vi "FFT Skew Detection.vi"(8 "error in (no error)":errorcluster, 11 "Refnum In":T2) -> (0 "error out":errorcluster, 1 "Error (Degrees)":dbl format="%_6g", 2 "Error (Radians)":dbl format="%_6f", 3 "Fit Line":T2(plugin-control), 4 "Alt. Angle (Degrees)":dbl format="%_6g", 5 "Alt. Angle (Radians)":dbl format="%_6g", 6 "Angle (Degrees)":dbl format="%_6g", 7 "Angle (Radians)":dbl format="%_6g")   [LabVIEW 2016]
uses:
  <vilib>/vision/Image Controls.llb/IMAQ Image.ctl
  <vilib>/Analysis/6fits.llb/Confidence Interval (Linear).vi
  <vilib>/vision/NI_Vision_Development_Module.lvlib
  <vilib>/Analysis/6fits.llb/Curve Fitting Criteria.ctl
  <vilib>/Analysis/NI_AALPro.lvlib
panel:
  in  "Tab Control":T1(tab)
  out "Original Image":T2(plugin-control)
  in  "File Path":path=path "D:/Documents/School/Brookhaven/Images/Pixel to Micron Test/image_000_600_60_15_rotated_45_degrees.png"
  out "FFT":T2(plugin-control)
  out "Zoom":T2(plugin-control)
  in  "Image Zoom":sgl=1.0
  out "Image Center Y":u32
  out "Image Center X":u32
  out "Captured FFT Spectrum":picture
  out "Load as U8":T2(plugin-control)
  in  "Settings":T3={"Objects"=0, "Threshold"=160, "Reject Border"=TRUE, "Fill Holes"=FALSE, "Min Object Size"=FALSE, "Min Size"=2, "Max Object Size"=FALSE, "Max Size"=100, "Show Search Area"=FALSE, "Show Center"=TRUE, "Show Bounding Box"=TRUE} {"Objects" items=["Bright Objects", "Dark Objects"]; "Threshold" min=1 max=999999999 step=1; "Max Size" min=1 max=999999999 step=1; "Min Size" min=1 max=999999999 step=1}
  out "Number of Objects Found":i32
  out "Find Objects":T2(plugin-control)
  out "Image Aspect Ratio":dbl
  out "Adjusted Slope Error":dbl format="%^_4e"
  out "Adjusted Slope":dbl format="%_6g"
  out "Line Equation":cluster{"A":dbl, "B":dbl, "C":dbl} {"C" format="%_6f"; "B" format="%_6f"; "A" format="%_6f"}
  out "Valid Fit?":bool
  out "X":sgl[](array[numeric])
  out "Y":sgl[](array[numeric])
  out "IMAQ Fit Slope":dbl format="%_6g"
  out "Residual":dbl format="%.2f"
  out "IMAQ Fit Intercept":dbl
  out "IMAQ Fit Delta Slope":dbl
  out "IMAQ Fit Delta Intercept":dbl
  out "Sigma":sgl[](array[numeric])
  # "Skew Angle (0 to 180 Degrees)"
  # "Skew Angle (90 to -90 Degrees)"
  # "Error"
  # "Line Fit"
  # "Ax + By + C = 0"
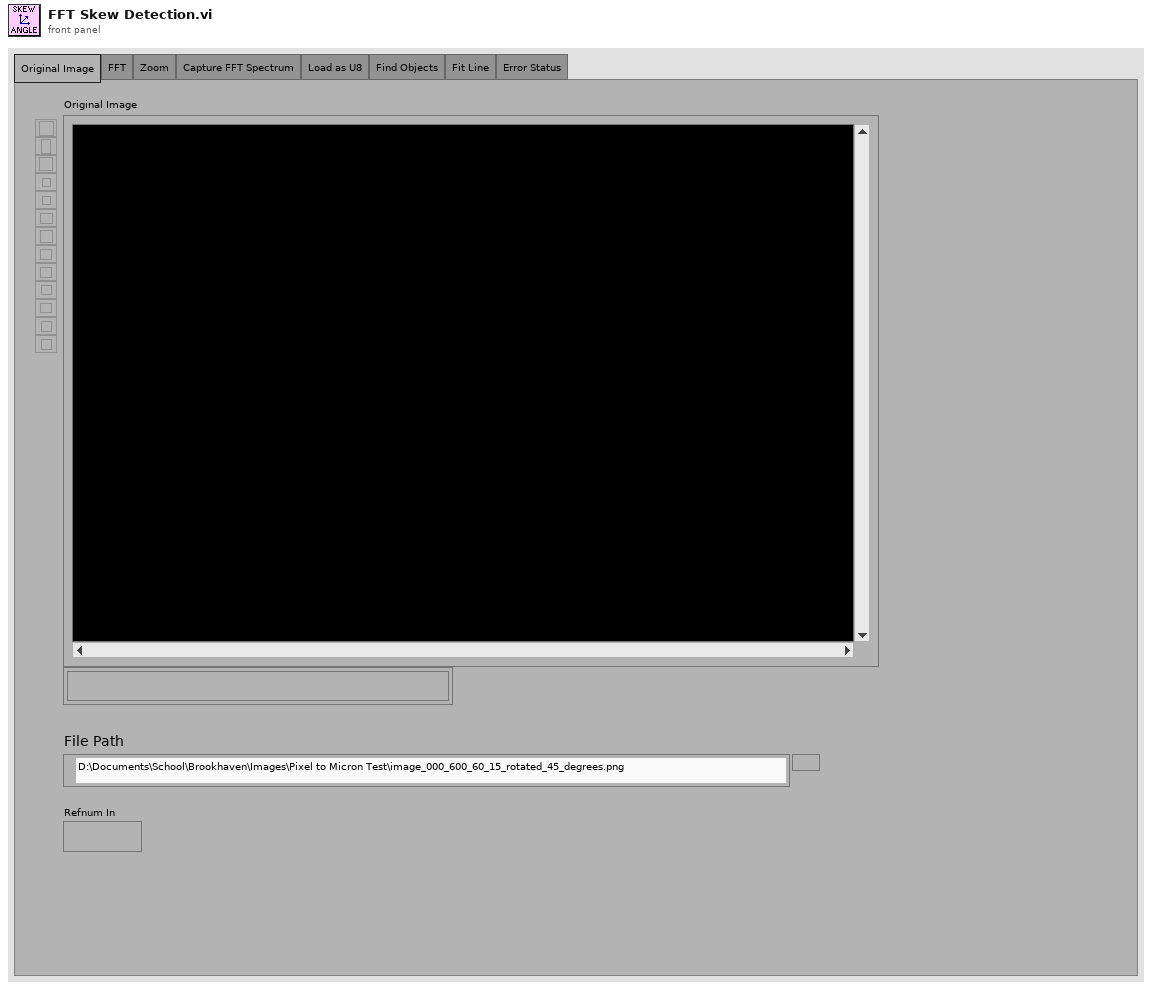
[diagram p1: front panel]
types:
  T1 = enum32{"Original Image", "FFT", "Zoom", "Capture FFT Spectrum", "Load as U8", "Find Objects", "Fit Line", "Error Status"}
  T2 = typedef "IMAQ Image.ctl" = refnum<image>
  T3 = cluster{"Objects":u16, "Threshold":i32, "Reject Border":bool, "Fill Holes":bool, "Min Object Size":bool, "Min Size":i32, "Max Object Size":bool, "Max Size":i32, "Show Search Area":bool, "Show Center":bool, "Show Bounding Box":bool}
  T4 = typedef "Image Type" = u32
  T5 = typedef "imagedata.ctl" = cluster{"image type":i32, "image depth":i32, "image":u8[], "mask":u8[], "colors":u32[], "Rectangle":cluster{"left":i16, "top":i16, "right":i16, "bottom":i16}}
  T6 = cluster{"Object Center":cluster{"X":sgl, "Y":sgl}, "Bounding Box":cluster{"X Left":i32, "Y Top":i32, "X Right":i32, "Y Bottom":i32}, "Area":sgl, "Orientation":sgl, "Aspect Ratio":sgl, "Nb Holes":i32}[]
  T7 = cluster{"Point 1":cluster{"X":sgl, "Y":sgl}, "Point 2":cluster{"X":sgl, "Y":sgl}}
  T8 = typedef "NI_AALPro.lvlib/Curve Fitting Criteria.ctl" = u16
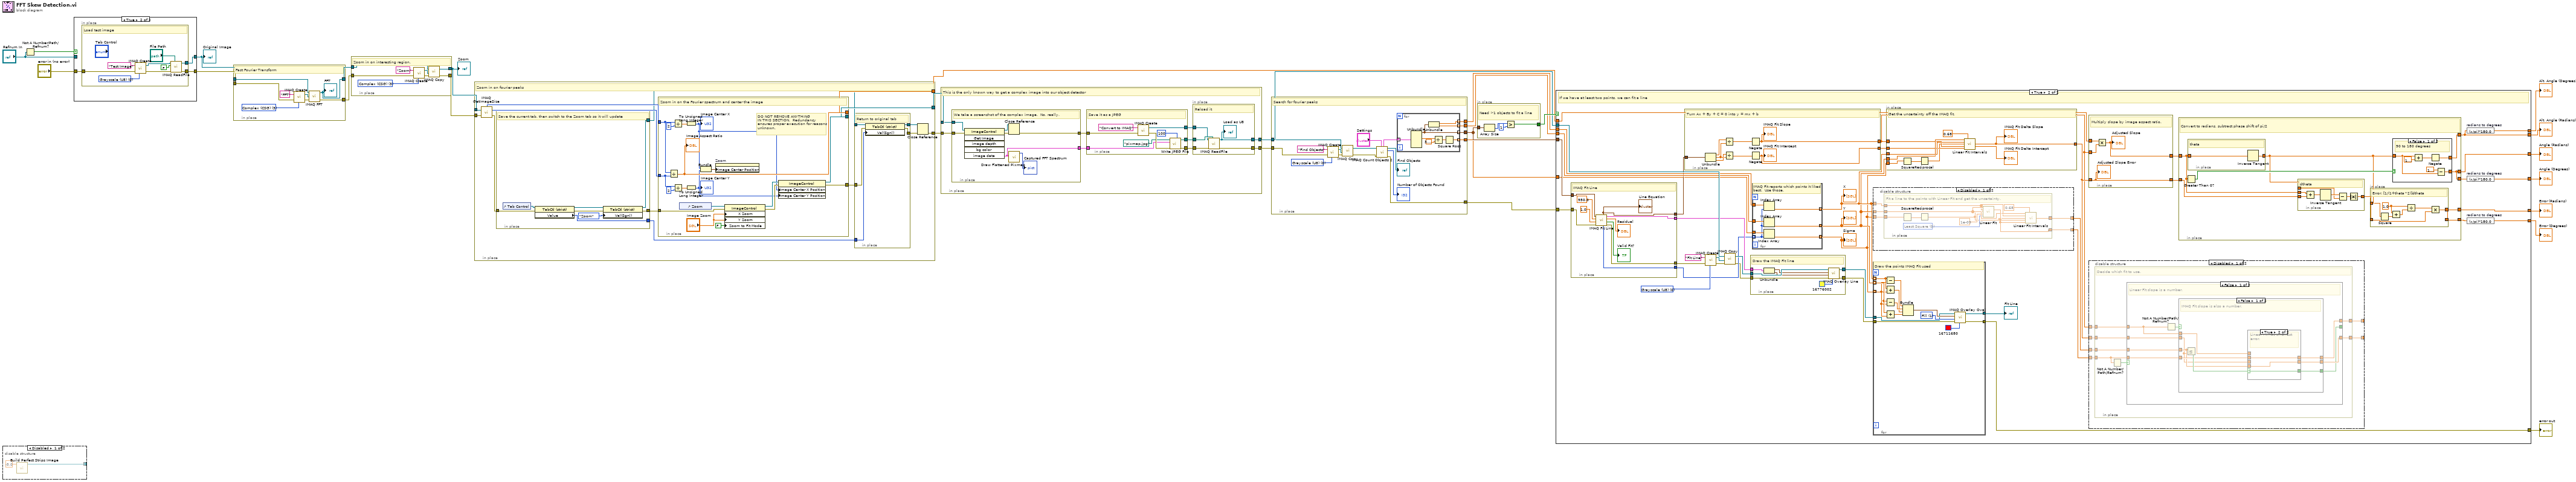
[diagram p0: block diagram]
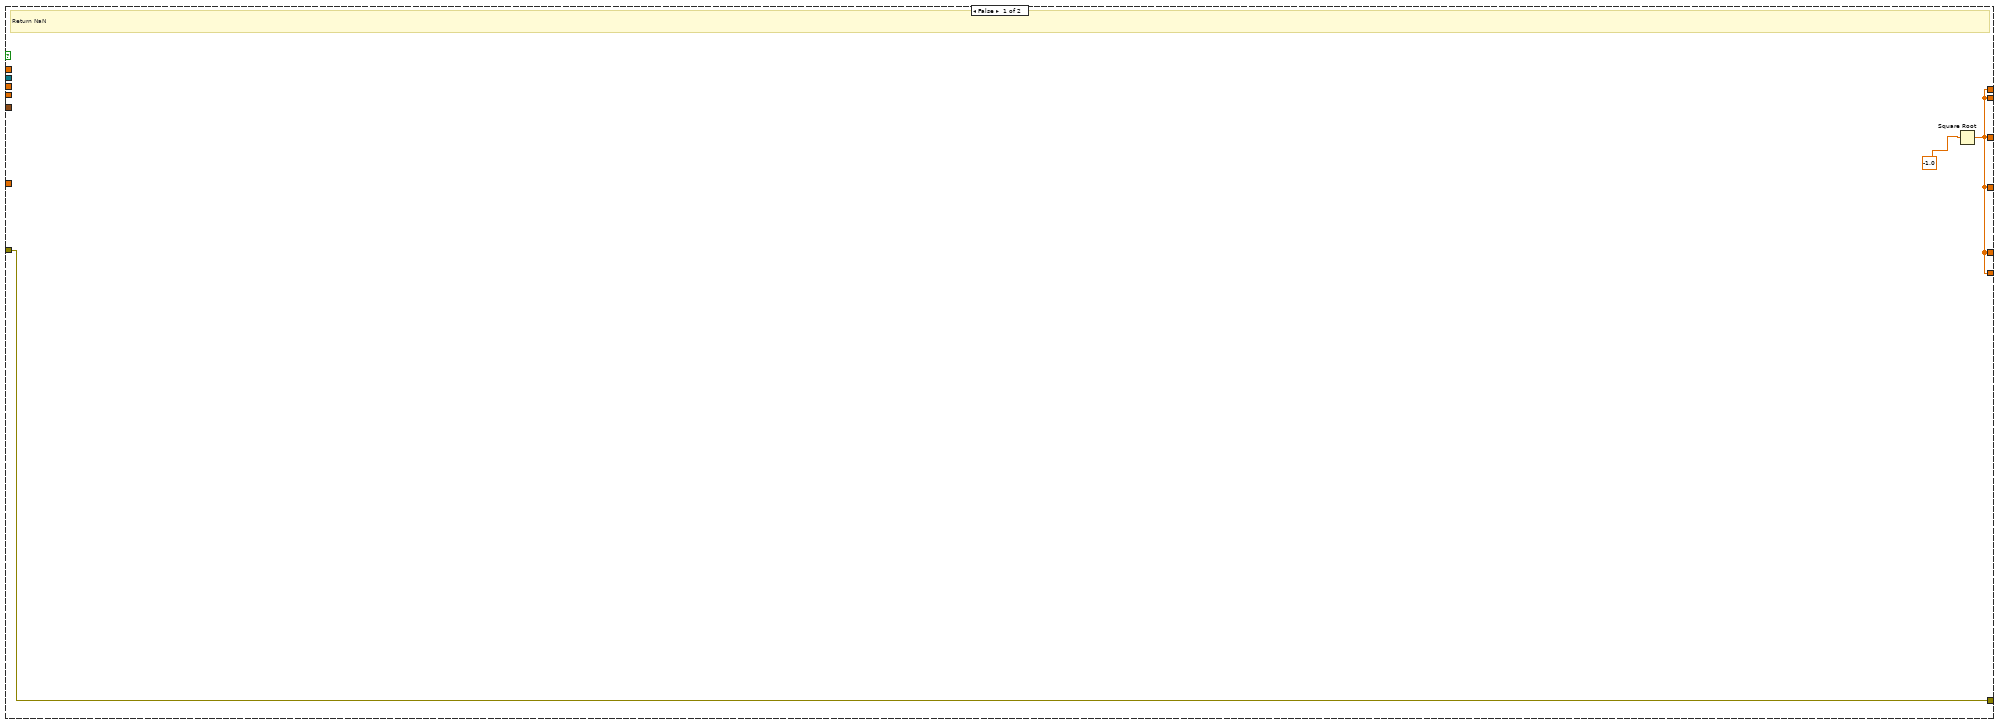
[diagram p4: hidden frame]
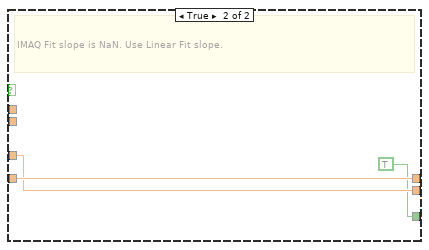
[diagram p7: hidden frame]
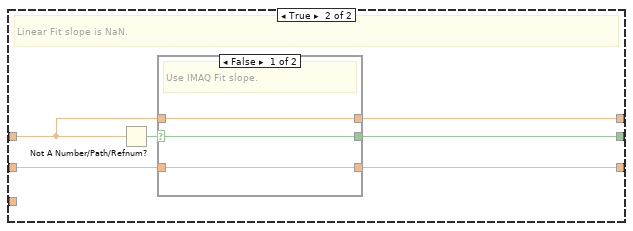
[diagram p8: hidden frame]
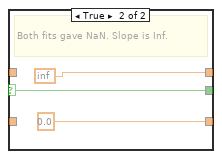
[diagram p9: hidden frame]
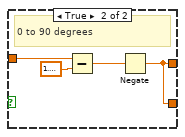
[diagram p11: hidden frame]
diagram:
  n1 = disable-structure shown="Disabled" {
    disable-tunnel: [w28 _] -> _
    frame Disabled {
      n2 = call "Build Perfect Strips Image.vi"("Angle (degrees)"=sgl -5.0) -> ("Image Out"=w28:T2)  [unwired: 9 in, 1 out]
    }
    frame Enabled {
    }
  }
  n3 = Not A Number/Path/Refnum?(number/path/refnum="Refnum In") -> (NaN/Path/Refnum?=w14:bool)
  n4 = case shown="True" w14 {
    tunnel: "error in (no error)" -> [w30 w34]
    tunnel: [w30 w33] -> w26
    tunnel: [w31 w32] -> w13
    tunnel: "Refnum In" -> [w31 _]
    frame False {
    }
    frame True {
      n5 = in-place {
        in-place-border: [w35] -> w32
        in-place-border: [w37] -> w33
        in-place-border: w34 -> [w36]
        w40 = T4 0 items=["Grayscale (U8)", "Grayscale (I16)", "Grayscale (SGL)", "Complex (CSG)", "RGB (U32)", "HSL (U32)", "RGB (U64)", "Grayscale (U16)"] ("Image Type")
        # "Load test image"
        n6 = call "IMAQ Create"("Image Name"="Test Image", "Image Type"=w40, "error in (no error)"=w36) -> ("New Image"=w41:T2, "error out"=w38:errorcluster)  [unwired: 2 in]
        n7 = call "IMAQ ReadFile"("File Path"="File Path", "error in (no error)"=w38, "Load Color Palette? (No)"=FALSE, "Image"=w41) -> ("error out"=w37:errorcluster, "Image Out"=w35:T2)  [unwired: 3 in, 3 out]
      }
    }
  }
  "Original Image" <- w13
  n8 = in-place {
    in-place-border: w26 -> [w51]
    in-place-border: w13 -> [w47]
    in-place-border: [w46] -> w22
    in-place-border: [w44] -> w8
    w49 = T4 3 items=["Grayscale (U8)", "Grayscale (I16)", "Grayscale (SGL)", "Complex (CSG)", "RGB (U32)", "HSL (U32)", "RGB (U64)", "Grayscale (U16)"] ("Image Type")
    # "Fast Fourier Transform"
    n9 = call "IMAQ Create"("Image Name"="FFT", "Image Type"=w49, "error in (no error)"=w51) -> ("New Image"=w48:T2, "error out"=w45:errorcluster)  [unwired: 2 in]
    n10 = call "IMAQ FFT"("error in (no error)"=w45, "Image Dst"=w48, "Image Src"=w47) -> ("error out"=w44:errorcluster, "Image Dst Out"=w46:T2)  [unwired: 1 in]
    "FFT" <- w46
  }
  n11 = in-place {
    in-place-border: w22 -> [w56]
    in-place-border: [w55] -> w10
    in-place-border: w8 -> [w54]
    in-place-border: [w52] -> w7
    w58 = T4 3 items=["Grayscale (U8)", "Grayscale (I16)", "Grayscale (SGL)", "Complex (CSG)", "RGB (U32)", "HSL (U32)", "RGB (U64)", "Grayscale (U16)"] ("Image Type")
    # "Zoom in on interesting region."
    n12 = call "IMAQ Create"("Image Name"="Zoom", "Image Type"=w58, "error in (no error)"=w54) -> ("New Image"=w57:T2, "error out"=w53:errorcluster)  [unwired: 2 in]
    n13 = call "IMAQ Copy"("error in (no error)"=w53, "Image Dst"=w57, "Image Src"=w56) -> ("error out"=w52:errorcluster, "Image Dst Out"=w55:T2)  [unwired: 3 in]
  }
  "Zoom" <- w10
  n14 = in-place {
    in-place-border: w10 -> [w73]
    in-place-border: [w70] -> w19
    in-place-border: [w69] -> w9
    in-place-border: w7 -> [w68]
    in-place-border: [w60] -> w6
    # "Zoom in on fourier peaks"
    n15 = call "IMAQ GetImageSize"("Image"=w73, "error in (no error)"=w68) -> ("Y Resolution"=w71:i32, "X Resolution"=w72:i32, "error out"=w66:errorcluster)  [unwired: 2 in]
    n16 = in-place {
      in-place-border: [w103] -> w67
      in-place-border: w66 -> [w101]
      in-place-border: [w98] -> w64
      in-place-border: [w97] -> w63
      # "Save the current tab, then switch to the Zoom tab so it will update"
      n17 = control-ref of="Tab Control"() -> (w102:refnum<vi>)
      n18 = property class="TabCtl (strict)"(reference=w102, error in=w101) -> (reference out=w99:refnum<vi>, error out=w100:errorcluster, "Value"=w97:T1)
      n19 = property class="TabCtl (strict)"(reference=w99, error in=w100, "Val(Sgnl)"=T1."Zoom" ("Value")) -> (reference out=w98:refnum<vi>, error out=w103:errorcluster)
    }
    n20 = in-place {
      in-place-border: w72 -> [w94]
      in-place-border: w71 -> [w93]
      in-place-border: [w92] -> w70
      in-place-border: [w87] -> w69
      in-place-border: w67 -> [w86]
      in-place-border: [w85] -> w65
      # "DO NOT REMOVE ANYTHING\nIN THIS SECTION.  Redundancy\nensures proper execution for reasons\nunknown."
      # "Zoom in on the Fourier spectrum and center the image"
      n21 = Divide(x=w94, y=w93) -> (x/y=w92:dbl)
      "Image Aspect Ratio" <- w92
      n22 = Divide(x=w94, y=2) -> (x/y=w91:dbl)
      n23 = Divide(x=w93, y=2) -> (x/y=w90:dbl)
      n24 = control-ref of="Zoom"() -> (w88:refnum<vi>)
      n25 = To Unsigned Long Integer(number=w91) -> (unsigned 32bit integer=w81:u32)
      "Image Center X" <- w81
      n26 = To Unsigned Long Integer(number=w90) -> (unsigned 32bit integer=w80:u32)
      "Image Center Y" <- w80
      n27 = Bundle(w81, w80) -> (w79:cluster{u32, u32})  [unwired: 1 in]
      n28 = property on="Zoom" class="ImageControl"("Image Center Position"=w79) -> ()  [unwired: 2 in, 2 out]
      n29 = property on="Property Node" class="ImageControl"(reference=w88, error in=w86, "X Zoom"="Image Zoom", "Y Zoom"="Image Zoom", "Zoom to Fit Mode"=FALSE) -> (reference out=w82:refnum<vi>, error out=w83:errorcluster)
      n30 = property on="Property Node" class="ImageControl"(reference=w82, error in=w83, "Image Center X Position"=w81, "Image Center Y Position"=w80) -> (reference out=w87:refnum<vi>, error out=w85:errorcluster)
    }
    n31 = in-place {
      in-place-border: w65 -> [w78]
      in-place-border: [w77] -> w61
      in-place-border: w64 -> [w76]
      in-place-border: w63 -> [w75]
      in-place-border: [w74] -> w62
      # "Return to original tab"
      n32 = property class="TabCtl (strict)"(reference=w76, error in=w78, "Val(Sgnl)"=w75) -> (reference out=w74:refnum<vi>, error out=w77:errorcluster)
    }
    n33 = Close Reference(reference=w62, error in (no error)=w61) -> (error out=w60:errorcluster)
  }
  n34 = in-place {
    in-place-border: [w109] -> w11
    in-place-border: w9 -> [w107]
    in-place-border: w6 -> [w106]
    in-place-border: [w105] -> w3
    # "This is the only known way to get a complex image into our object detector"
    n35 = in-place {
      in-place-border: [w133] -> w110
      in-place-border: [w128] -> w108
      in-place-border: w107 -> [w132]
      in-place-border: w106 -> [w131]
      # "We take a screenshot of the complex image.  No, really."
      n36 = invoke on="Invoke Node" class="ImageControl" method="Get Image"(reference=w132, error in=w131) -> (reference out=w130:refnum<vi>, error out=w129:errorcluster, "image data"=w133:T5)  [unwired: 4 in, 3 out]
      n37 = Close Reference(reference=w130, error in (no error)=w129) -> (error out=w128:errorcluster)
      n38 = call <vilib>:"Draw Flattened Pixmap.vi"("image data"=w133) -> ("new picture"=→"Captured FFT Spectrum":picture)  [unwired: 8 in]
    }
    n39 = in-place {
      in-place-border: [w127] -> w113
      in-place-border: [w126] -> w112
      in-place-border: [w124] -> w111
      in-place-border: w110 -> [w121]
      in-place-border: w108 -> [w119]
      # "Save it as a JPEG"
      n40 = call "IMAQ Create"("Image Name"="Convert to IMAQ", "error in (no error)"=w119) -> ("New Image"=w124:T2, "error out"=w123:errorcluster)  [unwired: 2 in, 1 out]
      n41 = call <vilib>:"Write JPEG File.vi"("quality (80)"=100, "error in (no error)"=w123, "image data"=w121, "path to JPEG file"=path "pixmap.jpg") -> ("error out"=w126:errorcluster, "path"=w127:path)  [unwired: 6 out]
    }
    n42 = in-place {
      in-place-border: w113 -> [w118]
      in-place-border: w112 -> [w117]
      in-place-border: w111 -> [w116]
      in-place-border: [w115] -> w109
      in-place-border: [w114] -> w105
      # "Reload it"
      n43 = call "IMAQ ReadFile"("File Path"=w118, "error in (no error)"=w117, "Image"=w116) -> ("error out"=w114:errorcluster, "Image Out"=w115:T2)  [unwired: 2 in, 5 out]
      "Load as U8" <- w115
    }
  }
  n44 = in-place {
    in-place-border: [w148] -> w12
    in-place-border: [w147] -> w24
    in-place-border: [w146] -> w23
    in-place-border: w11 -> [w145]
    in-place-border: [w139] -> w5
    in-place-border: [w138] -> w4
    in-place-border: w3 -> [w135]
    w141 = T4 0 items=["Grayscale (U8)", "Grayscale (I16)", "Grayscale (SGL)", "Complex (CSG)", "RGB (U32)", "HSL (U32)", "RGB (U64)", "Grayscale (U16)"] ("Image Type")
    # "Search for fourier peaks"
    n45 = call "IMAQ Create"("Image Name"="Find Objects", "Image Type"=w141, "error in (no error)"=w135) -> ("New Image"=w140:T2, "error out"=w136:errorcluster)  [unwired: 2 in]
    n46 = call "IMAQ Copy"("error in (no error)"=w136, "Image Dst"=w140, "Image Src"=w145) -> ("error out"=w137:errorcluster, "Image Dst Out"=w144:T2)  [unwired: 3 in]
    n47 = call "IMAQ Count Objects 2"("Settings"="Settings", "error in (no error)"=w137, "Image"=w144) -> ("error out"=w138:errorcluster, "Number of Objects"=→"Number of Objects Found":i32, "Image Out"=→"Find Objects":T2, "Objects"=w150:T6)  [unwired: 4 in, 1 out]
    n48 = for {
      tunnel: w150 -> [w159] mode=indexing
      tunnel: [w158] -> w147 mode=indexing
      tunnel: [w157] -> w146 mode=indexing
      tunnel: [w156] -> w148 mode=indexing
      tunnel: [w155] -> w139 mode=indexing
      n49 = Unbundle(w159) -> ("Object Center"=w156:cluster{"X":sgl, "Y":sgl}, "Area"=w154:sgl)  [unwired: 4 out]
      n50 = Unbundle(w156) -> ("X"=w158:sgl, "Y"=w157:sgl)
      n51 = Divide(x=w154, y=3.141592653589793) -> (x/y=w152:dbl)
      n52 = Square Root(x=w152) -> (sqrt(x)=w155:dbl)
    }
  }
  n53 = in-place {
    in-place-border: w12 -> [w163]
    in-place-border: [w160] -> w25
    # "Need >1 objects to fit a line"
    n54 = Array Size(array=w163) -> (size(s)=w162:i32)
    n55 = Greater?(x=w162, y=1) -> (0:w160:bool)
  }
  n56 = case shown="True" w25 {
    tunnel: w24 -> [_ w186]
    tunnel: w23 -> [_ w185]
    tunnel: w19 -> [_ w176]
    tunnel: [w165 w203] -> w21
    tunnel: [w165 w202] -> w20
    tunnel: [w165 w201] -> w18
    tunnel: [w165 w200] -> w17
    tunnel: [w165 w198] -> w16
    tunnel: [w165 w197] -> w15
    tunnel: w12 -> [_ w196]
    tunnel: w11 -> [_ w192]
    tunnel: w5 -> [_ w171]
    tunnel: [w164 w183] -> w2
    tunnel: w4 -> [w164 w178]
    frame False {
      # "Return NaN"
      n57 = Square Root(x=-1.0) -> (sqrt(x)=w165:dbl)
    }
    frame True {
      w194 = T4 0 items=["Grayscale (U8)", "Grayscale (I16)", "Grayscale (SGL)", "Complex (CSG)", "RGB (U32)", "HSL (U32)", "RGB (U64)", "Grayscale (U16)"] ("Image Type")
      # "If we have at least two points, we can fit a line"
      n58 = in-place {
        in-place-border: w196 -> [w301]
        in-place-border: [w298] -> w191
        in-place-border: [w297] -> w187
        in-place-border: [w296] -> w184
        in-place-border: [w294] -> w179
        in-place-border: w178 -> [w293]
        # "IMAQ Fit Line"
        n59 = call "IMAQ Fit Line"("error in (no error)"=w293, "Pixel Radius"=sgl 1.0, "Minimum Score"=sgl 950.0, "Points"=w301) -> ("error out"=w294:errorcluster, "Valid Fit?"=→"Valid Fit?":bool, "Residual"=→"Residual":dbl, "Line Segment"=w298:T7, "Indexes of Points Used"=w297:i32[], "Line Equation"=w296:cluster{"A":dbl, "B":dbl, "C":dbl})  [unwired: 2 in]
        "Line Equation" <- w296
      }
      n60 = in-place {
        in-place-border: w184 -> [w281]
        in-place-border: [w274] -> w177
        in-place-border: [w275] -> w167
        # "Turn Ax + By + C = 0 into y = mx + b"
        n61 = Unbundle(w281) -> ("A"=w280:dbl, "B"=w277:dbl, "C"=w278:dbl)
        n62 = Divide(x=w280, y=w277) -> (x/y=w279:dbl)
        n63 = Divide(x=w278, y=w277) -> (x/y=w276:dbl)
        n64 = Negate(x=w279) -> (-x=w275:dbl)
        "IMAQ Fit Slope" <- w275
        n65 = Negate(x=w276) -> (-x=w274:dbl)
        "IMAQ Fit Intercept" <- w274
      }
      n66 = call "IMAQ Create"("Image Name"="Fit Line", "Image Type"=w194, "error in (no error)"=w179) -> ("New Image"=w193:T2, "error out"=w180:errorcluster)  [unwired: 2 in]
      n67 = call "IMAQ Copy"("error in (no error)"=w180, "Image Dst"=w193, "Image Src"=w192) -> ("error out"=w181:errorcluster, "Image Dst Out"=w190:T2)  [unwired: 3 in]
      n68 = in-place {
        in-place-border: w190 -> [w316]
        in-place-border: w191 -> [w315]
        in-place-border: [w311] -> w189
        in-place-border: [w310] -> w182
        in-place-border: w181 -> [w309]
        # "Draw the IMAQ Fit line"
        n69 = Unbundle(w315) -> ("Point 1"=w314:cluster{"X":sgl, "Y":sgl}, "Point 2"=w313:cluster{"X":sgl, "Y":sgl})
        n70 = call "IMAQ Overlay Line"("Color"=u32 16776002, "error in (no error)"=w309, "End Point"=w313, "Start Point"=w314, "Image"=w316) -> ("error out"=w310:errorcluster, "Image Out"=w311:T2)  [unwired: 5 in]
      }
      n71 = for {
        tunnel: w187 -> [w303] mode=indexing
        tunnel: w186 -> [w308]
        tunnel: w185 -> [w307]
        tunnel: [w306] -> w173 mode=indexing
        tunnel: [w305] -> w172 mode=indexing
        tunnel: w171 -> [w304]
        tunnel: [w302] -> w169 mode=indexing
        # "IMAQ Fit reports which points it liked best.  Use those."
        n72 = Index Array(array=w308, index=w303) -> (element=w306:sgl)
        n73 = Index Array(array=w307, index=w303) -> (element=w305:sgl)
        n74 = Index Array(array=w304, index=w303) -> (element=w302:dbl)
      }
      "X" <- w173
      "Y" <- w172
      "Sigma" <- w169
      n75 = disable-structure shown="Disabled" {
        disable-tunnel: [w210 _] -> w175
        disable-tunnel: [w209 _] -> w174
        disable-tunnel: w173 -> [w208 _]
        disable-tunnel: w172 -> [w207 _]
        disable-tunnel: w169 -> [w206 _]
        frame Disabled {
          n76 = in-place {
            in-place-border: w208 -> [w219]
            in-place-border: w207 -> [w220]
            in-place-border: w206 -> [w218]
            in-place-border: [w221] -> w209
            in-place-border: [w222] -> w210
            w217 = T8 0 items=["Least Square", "Least Absolute Residual", "Bisquare"] ("method")
            # "Fit a line to the points with Linear Fit and get the uncertainty."
            n77 = Square(x=w218) -> (x^2=w212:dbl[])
            n78 = Reciprocal(x=w212) -> (1/x=w211:dbl[])
            n79 = call <vilib>:"Linear Fit.vi"("Y"=w220, "X"=w219, "Weight"=w211, "tolerance"=1e-09, "method"=w217) -> ("slope"=w222:dbl, "intercept"=w215:dbl)  [unwired: 6 in, 3 out]
            n80 = call-poly <vilib>:"Linear Fit Intervals.vi"("Y"=w220, "confidence level"=0.68, "X"=w219, "Weight"=w211, "slope"=w222, "intercept"=w222) -> ("delta slope"=w221:dbl, "delta intercept"=w213:dbl)  [unwired: 5 in, 3 out]
          }
        }
        frame Enabled {
        }
      }
      n81 = for {
        tunnel: w173 -> [w330] mode=indexing
        tunnel: w172 -> [w329] mode=indexing
        tunnel: w189 -> [w322]
        tunnel: [w321] -> w188
        tunnel: [w319] -> w183
        tunnel: w182 -> [w318]
        tunnel: w169 -> [w317] mode=indexing
        w323 = u32 1 items=["Frame", "Fill"] ("Drawing Mode (Frame)")
        # "Draw the points IMAQ Fit used"
        n82 = Subtract(x=w330, y=w317) -> (x-y=w328:dbl)
        n83 = Add(x=w330, y=w317) -> (x+y=w326:dbl)
        n84 = Subtract(x=w329, y=w317) -> (x-y=w327:dbl)
        n85 = Add(x=w329, y=w317) -> (x+y=w325:dbl)
        n86 = Bundle(w328, w327, w326, w325) -> (w324:cluster{dbl, dbl, dbl, dbl})  [unwired: 1 in]
        n87 = call "IMAQ Overlay Oval"("Color"=u32 16711680, "error in (no error)"=w318, "Drawing Mode (Frame)"=w323, "Bounding Rectangle"=w324, "Image"=w322) -> ("error out"=w319:errorcluster, "Image Out"=w321:T2)  [unwired: 5 in]
      }
      "Fit Line" <- w188
      n88 = in-place {
        in-place-border: [w286] -> w168
        in-place-border: w173 -> [w290]
        in-place-border: w172 -> [w289]
        in-place-border: w169 -> [w283]
        in-place-border: w167 -> [w288]
        in-place-border: w177 -> [w287]
        # "Get the uncertainty off the IMAQ fit."
        n89 = Square(x=w283) -> (x^2=w284:dbl[])
        n90 = Reciprocal(x=w284) -> (1/x=w282:dbl[])
        n91 = call-poly <vilib>:"Linear Fit Intervals.vi"("Y"=w289, "confidence level"=0.68, "X"=w290, "Weight"=w282, "slope"=w288, "intercept"=w287) -> ("delta slope"=w286:dbl, "delta intercept"=→"IMAQ Fit Delta Intercept":dbl)  [unwired: 5 in, 3 out]
        "IMAQ Fit Delta Slope" <- w286
      }
      n92 = disable-structure shown="Disabled" {
        disable-tunnel: w167 -> [w228 _]
        disable-tunnel: w168 -> [w227 _]
        disable-tunnel: w175 -> [w226 _]
        disable-tunnel: w174 -> [w225 _]
        disable-tunnel: [w224 _] -> _
        disable-tunnel: [w223 _] -> _
        frame Disabled {
          n93 = in-place {
            in-place-border: w228 -> [w235]
            in-place-border: w227 -> [w234]
            in-place-border: w226 -> [w233]
            in-place-border: w225 -> [w232]
            in-place-border: [w231] -> w224
            in-place-border: [w230] -> w223
            # "Decide which fit to use."
            n94 = Not A Number/Path/Refnum?(number/path/refnum=w233) -> (NaN/Path/Refnum?=w236:bool)
            n95 = case shown="False" w236 {
              tunnel: w235 -> [w238 w264]
              tunnel: [w242 w266] -> w231
              tunnel: [w240 w265] -> w230
              tunnel: w234 -> [w239 w263]
              tunnel: w233 -> [w243 _]
              tunnel: w232 -> [w241 _]
              tunnel: [w237 w262] -> w229
              frame False {
                # "Linear Fit slope is a number."
                n96 = Not A Number/Path/Refnum?(number/path/refnum=w238) -> (NaN/Path/Refnum?=w244:bool)
                n97 = case shown="False" w244 {
                  tunnel: [w250 w261] -> w242
                  tunnel: [w248 w260] -> w240
                  tunnel: w243 -> [w251 w261]
                  tunnel: w241 -> [w249 w260]
                  tunnel: w239 -> [w246 _]
                  tunnel: w238 -> [w247 _]
                  tunnel: [w245 TRUE] -> w237
                  frame False {
                    # "IMAQ Fit slope is also a number."
                    n98 = Less Or Equal?(x=w249, y=w246) -> (x <= y?=w252:bool)
                    n99 = case shown="True" w252 {
                      selector: w252 -> [w253 w256]
                      tunnel: w251 -> [_ w258]
                      tunnel: [w255 w258] -> w250
                      tunnel: w249 -> [_ w257]
                      tunnel: [w254 w257] -> w248
                      tunnel: w247 -> [w255 _]
                      tunnel: w246 -> [w254 _]
                      tunnel: [w253 w256] -> w245
                      frame False {
                        # "IMAQ Fit has smallest error."
                      }
                      frame True {
                        # "Linear Fit has smallest error."
                      }
                    }
                  }
                  frame True {
                    # "IMAQ Fit slope is NaN. Use Linear Fit slope."
                  }
                }
              }
              frame True {
                # "Linear Fit slope is NaN."
                n100 = Not A Number/Path/Refnum?(number/path/refnum=w264) -> (NaN/Path/Refnum?=w267:bool)
                n101 = case shown="False" w267 {
                  selector: w267 -> [w268 w271]
                  tunnel: [w270 inf] -> w266
                  tunnel: [w269 0.0] -> w265
                  tunnel: w264 -> [w270 _]
                  tunnel: w263 -> [w269 _]
                  tunnel: [w268 w271] -> w262
                  frame False {
                    # "Use IMAQ Fit slope."
                  }
                  frame True {
                    # "Both fits gave NaN. Slope is Inf."
                  }
                }
              }
            }
          }
        }
        frame Enabled {
        }
      }
      n102 = in-place {
        in-place-border: w176 -> [w369]
        in-place-border: [w368] -> w205
        in-place-border: w167 -> [w367]
        in-place-border: w168 -> [w366]
        in-place-border: [w366] -> w170
        # "Multiply slope by image aspect ratio."
        n103 = Multiply(x=w369, y=w367) -> (x*y=w368:dbl)
        "Adjusted Slope" <- w368
        "Adjusted Slope Error" <- w366
      }
      n104 = in-place {
        in-place-border: w205 -> [w334]
        in-place-border: [w339] -> w204
        in-place-border: [w339] -> w202
        in-place-border: [w337] -> w201
        in-place-border: [w336] -> w199
        in-place-border: [w335] -> w198
        in-place-border: w170 -> [w331]
        # "Convert to radians, subtract phase shift of pi/2"
        n105 = Greater Than 0?(x=w334) -> (x > 0?=w338:bool)
        n106 = in-place {
          in-place-border: w334 -> [w348]
          in-place-border: [w347] -> w333
          # "theta"
          n107 = Inverse Tangent(1:w348) -> (0:w347:dbl)
        }
        n108 = in-place {
          in-place-border: w334 -> [w343]
          in-place-border: w333 -> [w342]
          in-place-border: [w341] -> w332
          in-place-border: w331 -> [w340]
          # "dtheta"
          n109 = Add(x=w343, y=w340) -> (x+y=w344:dbl)
          n110 = Inverse Tangent(1:w344) -> (0:w345:dbl)
          n111 = Subtract(x=w345, y=w342) -> (x-y=w346:dbl)
          n112 = Absolute Value(x=w346) -> (abs(x)=w341:dbl)
        }
        n113 = in-place {
          in-place-border: w333 -> [w354]
          in-place-border: [w350] -> w336
          in-place-border: [w350] -> w335
          in-place-border: w332 -> [w349]
          w355 = 1.0
          # "Error: [1/(1+theta^2)]dtheta"
          n114 = Square(x=w354) -> (x^2=w353:dbl)
          n115 = Add(x=w355, y=w353) -> (x+y=w352:dbl)
          n116 = Divide(x=w355, y=w352) -> (x/y=w351:dbl)
          n117 = Multiply(x=w351, y=w349) -> (x*y=w350:dbl)
        }
        n118 = case shown="False" w338 {
          tunnel: w333 -> [w357 w364]
          tunnel: [w360 w362] -> w339
          tunnel: [w356 w362] -> w337
          frame False {
            # "90 to 180 degrees"
            n119 = Add(x=w357, y=1.5707963267948966) -> (x+y=w358:dbl)
            n120 = Negate(x=w358) -> (-x=w356:dbl)
            n121 = Subtract(x=1.5707963267948966, y=w357) -> (x-y=w360:dbl)
          }
          frame True {
            # "0 to 90 degrees"
            n122 = Subtract(x=w364, y=1.5707963267948966) -> (x-y=w363:dbl)
            n123 = Negate(x=w363) -> (-x=w362:dbl)
          }
        }
      }
      n124 = expression code="(x/pi)*180.0" "radians to degrees"(w201) -> (w200:dbl)
      n125 = expression code="(x/pi)*180.0" "radians to degrees"(w204) -> (w203:dbl)
      n126 = expression code="(x/pi)*180.0" "radians to degrees"(w199) -> (w197:dbl)
    }
  }
  "Angle (Radians)" <- w20
  "Angle (Degrees)" <- w21
  "Alt. Angle (Radians)" <- w18
  "Alt. Angle (Degrees)" <- w17
  "Error (Radians)" <- w16
  "Error (Degrees)" <- w15
  "error out" <- w2
